vi "Send Settings.vi"(8 "error in":errorcluster, 11 "4124 in":refnum<class "4124.lvclass">) -> (0 "error out":errorcluster, 3 "4124 out":refnum<class "4124.lvclass">)   [LabVIEW 2018, in "4124.lvlib" / "4124.lvclass"]
uses:
  4124.lvclass
  <instrlib>/NI RMX-412x Power Supplies/NI RMX-412x Power Supplies.lvlib
  builds/Power_Supply.lvlibp/Power Supply.lvclass
  C:/Users/Ron.Dexter.LUMINARTECH/Desktop/builds/Power_Supply.lvlibp/Power Supply.lvclass
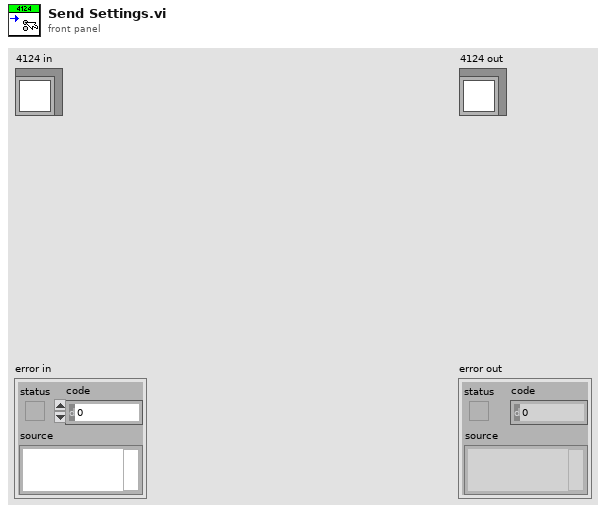
[diagram p1: front panel]
types:
  T1 = typedef "Power_Supply.lvlibp/Supply Settings.ctl" = cluster{"Voltage":dbl, "Current":dbl, "Output":bool}
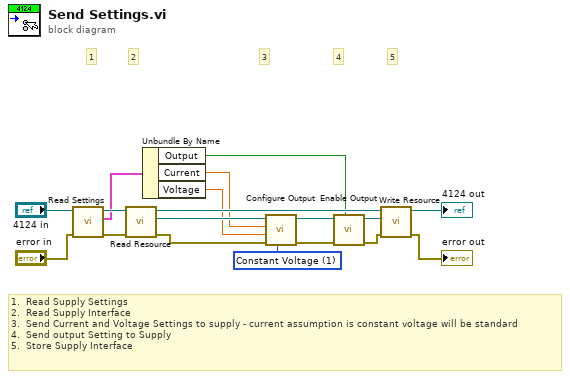
[diagram p0: block diagram]
diagram:
  w18 = 1 items=["Constant Current", "Constant Voltage"] ("Operation Mode (0: Constant Current)")
  # "1.  Read Supply Settings\n2.  Read Supply Interface\n3.  Send Current and Voltage Settings to supply - current assumption is constant voltage will be standard\n4.  Send output Setting to Supply\n5.  Store Supply Interface"
  # "5"
  # "4"
  # "3"
  # "2"
  # "1"
  n1 = call "Read Settings.vi"("error in (no error)"="error in", "Power Supply in"="4124 in") -> ("error out"=w15:errorcluster, "Settings"=w7:T1, "Power Supply out"=w16:refnum<class "4124.lvclass">)  [unwired: 7 in]
  n2 = call "Read Resource.vi"("error in"=w15, "Power Supply in"=w16) -> ("error out"=w10:errorcluster, "Resource"=w13:refnum<visa-resource-name>, "Power Supply out"=w14:refnum<class "4124.lvclass">)  [unwired: 7 in]
  n3 = Unbundle By Name(w7) -> ("Output"=w4:bool, "Current"=w5:dbl, "Voltage"=w6:dbl)
  n4 = call <instrlib>:"Configure Output.vi"("Operation Mode (0: Constant Current)"=w18, "error in (no error)"=w10, "Output Voltage (0 V)"=w6, "Output Current (0 A)"=w5, "VISA resource name"=w13) -> ("error out"=w9:errorcluster, "VISA resource name out"=w12:refnum<visa-resource-name>)  [unwired: 5 in]
  n5 = call <instrlib>:"Enable Output.vi"("Enable Output (F: Disable)"=w4, "error in (no error)"=w9, "VISA resource name"=w12) -> ("error out"=w8:errorcluster, "VISA resource name out"=w11:refnum<visa-resource-name>)  [unwired: 7 in]
  n6 = call "Write Resource.vi"("error in"=w8, "Resource"=w11, "Power Supply in"=w14) -> ("error out"=→"error out":errorcluster, "Power Supply out"=→"4124 out":refnum<class "4124.lvclass">)  [unwired: 7 in]
